vi "max and min.vi"() -> ()   [LabVIEW 2023]
panel:
  out "min":dbl
  out "max":dbl
  in  "array":dbl[](array[numeric])
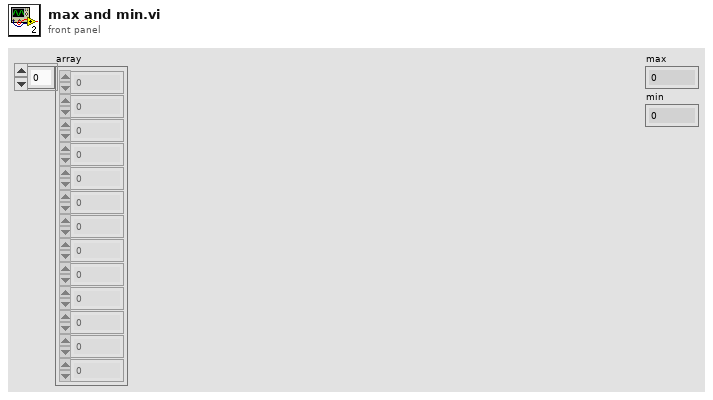
[diagram p1: front panel]
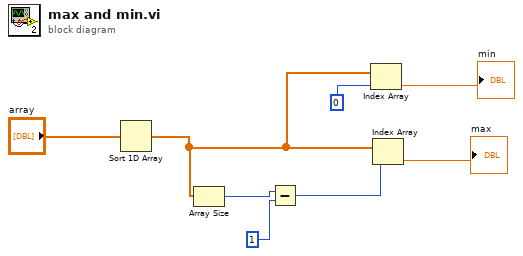
[diagram p0: block diagram]
diagram:
  n1 = Sort 1D Array(array="array") -> (sorted array=w3:dbl[])
  n2 = Array Size(array=w3) -> (size(s)=w7:i32)
  n3 = Subtract(x=w7, y=1) -> (x-y=w5:i32)
  n4 = Index Array(array=w3, index=0) -> (element=→"min":dbl)
  n5 = Index Array(array=w3, index=w5) -> (element=→"max":dbl)
